vi "Simple Add.vi"() -> ()   [LabVIEW 2017]
panel:
  out "x+y":i32
  in  "Numeric 2":i32
  in  "Numeric":i32
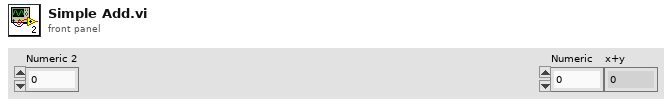
[diagram p1: front panel]
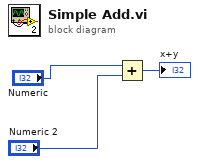
[diagram p0: block diagram]
diagram:
  n1 = Add(x="Numeric", y="Numeric 2") -> (x+y=→"x+y":i32)
